vi "CONTROL_SIGN.vi"(0 "VISA IN":refnum<visa-resource-name>, 5 "error in":errorcluster, 7 "Channel":i32) -> (14 "VISA Out":refnum<visa-resource-name>, 19 "error out":errorcluster)   [LabVIEW 2018, in "PNA-X.lvlib"]
doc: "CONTROL:SIGNal <conn>) \nParameters \n<ch> Any existing channel number. If unspecified, value is set to 1. \n<char> Choose from: \nMAIN - meas trig ready \nMATH - material handler \nAUXT - auxio (PNA-L and E836xB ONLY) \nExamples TRIG:CHAN:ROUT:INP MAIN \ntrigger:channel2:route:input main \nQuery Syntax TRIGger:CHANnel<ch>:ROUTe:INPut? \nReturn Type Character \nDefault \nTRIGger:CHANnel<ch>:ROUTe:READy <char> \n(Read-Write) Specifies the connector to use for the external trigger OUT ready line. \nParameters \n<ch> Any existing channel number. If unspecified, value is set to 1. \n<char> Choose from: \nMAIN - Meas trig ready \nMATH - Material handler pin 21 \nAUXT - AUX I/O pin 18 (PNA-L and E836xB ONLY) \nExamples TRIG:CHAN:ROUT:READ main \ntrigger:channel2:route:ready auxt \nQuery Syntax TRIGger:CHANnel<ch>:ROUTe:READy? \nReturn Type Character \nDefault"
uses:
  PNA-X.lvlib
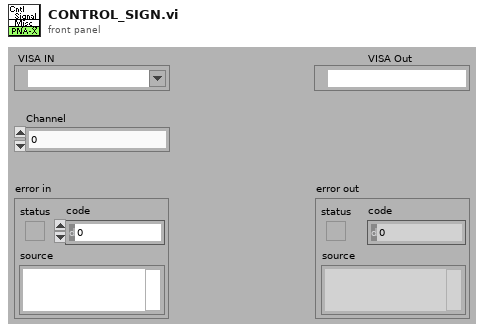
[diagram p1: front panel]
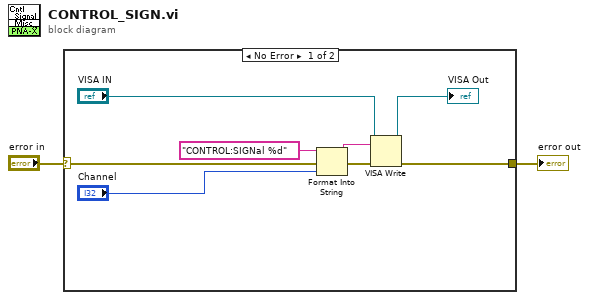
[diagram p0: block diagram]
diagram:
  n1 = case shown="No Error" "error in" {
    selector: "error in" -> [w10 w11]
    tunnel: [w5 w11] -> w1
    frame No Error {
      n2 = Format Into String(format string="CONTROL:SIGNal %d" ("Cmdline"), error in=w10, "Channel") -> (resulting string=w8:string, error out=w9:errorcluster)  [unwired: 1 in]
      n3 = VISA Write(VISA resource name="VISA IN", write buffer=w8, error in (no error)=w9) -> (VISA resource name out=→"VISA Out":refnum<visa-resource-name>, error out=w5:errorcluster)  [unwired: 1 out]
    }
    frame Error {
    }
  }
  "error out" <- w1
